vi "Create New Test Report.vi"(8 "error in":errorcluster, 10 "Test Name":string, 11 "Launcher in":refnum<class "Launcher.lvclass">) -> (0 "error out":errorcluster, 3 "Launcher out":refnum<class "Launcher.lvclass">)   [LabVIEW 2023, in "Launcher.lvlib" / "Launcher.lvclass"]
uses:
  Library/Launcher.lvclass
  Library/Launcher.lvclass/Launcher.ctl
  builds/Base Software/Base Software.lvlibp/Base Software Messages/Automation Update Test Name Msg/Automation Update Test Name Msg.lvclass
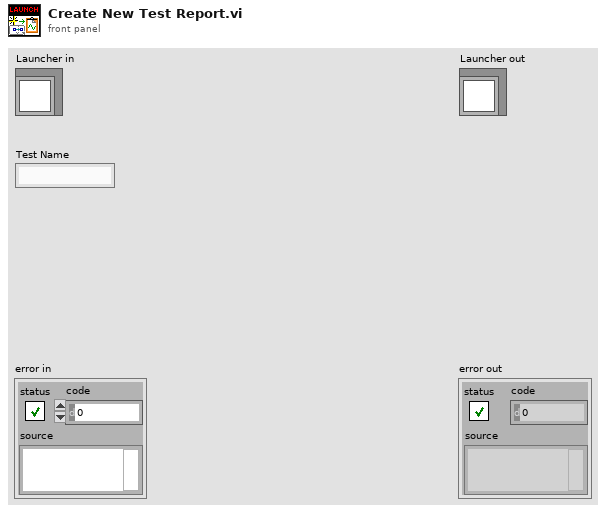
[diagram p1: front panel]
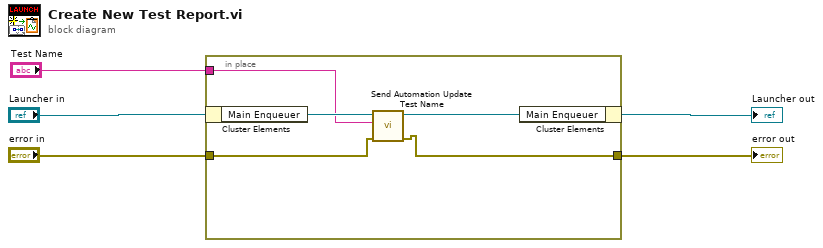
[diagram p0: block diagram]
diagram:
  n1 = in-place {
    in-place-border: "Test Name" -> [w8]
    in-place-border: "error in" -> [w7]
    in-place-border: [w6] -> w1
    n2 = in-place-cluster #1("Launcher in") -> ("Main Enqueuer"=w10:refnum<class "Message Enqueuer.lvclass">)
    n3 = call "Send Automation Update Test Name.vi"("error in (no error)"=w7, "Test Name"=w8, "Message Enqueuer"=w10) -> ("error out"=w6:errorcluster, "Message Enqueuer out"=w9:refnum<class "Message Enqueuer.lvclass">)  [unwired: 7 in]
    n4 = in-place-cluster #1("Main Enqueuer"=w9) -> (→"Launcher out":refnum<class "Launcher.lvclass">)
  }
  "error out" <- w1
